vi "Actor Core.vi"(8 "error in":errorcluster, 11 "Counter in":refnum<class "Counter.lvclass">) -> (0 "error out":errorcluster, 3 "Actor out":refnum<class "Actor.lvclass">)   [LabVIEW 2013, in "Counter.lvclass"]
doc: "(<B>Filename</B>: Actor Framework.lvlib:Actor.lvclass:Actor Core.vi)\n\nReceives messages to the actor, reacts to them, and initiates any error handling that may shut the actor down.\n\nDescendant classes may override this VI to append parallel tasks for the actor to complete while it handles messages. Overrides use the Call Parent Method node."
uses:
  Counter.lvclass
  <vilib>/ActorFramework/Actor/Actor.lvclass
  Display.lvclass/DisplayUI.lvclass
  <vilib>/ActorFramework/Actor/Actor.lvclass/Actor.ctl
  <vilib>/ActorFramework/Message Enqueuer/Message Enqueuer.lvclass/Message Enqueuer.ctl
  Counter.lvclass/Counter.ctl
  <vilib>/ActorFramework/Message Enqueuer/Init from Existing Queue.vi
  <vilib>/ActorFramework/Message Enqueuer/Enqueue.vi
  <vilib>/ActorFramework/Message Priority Queue/Priority Enqueue.vi
  <vilib>/ActorFramework/Message Enqueuer/Message Enqueuer.lvclass
  <vilib>/ActorFramework/Stop Msg/Stop Msg.lvclass
  Counter Messages/CountZero Msg/CountZero Msg.lvclass
  Counter Messages/DataToDisplay Msg/DataToDisplay Msg.lvclass
panel:
  in  "ToZero":bool
  in  "Exit":bool
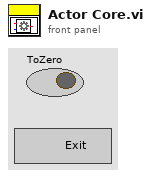
[diagram p1: front panel]
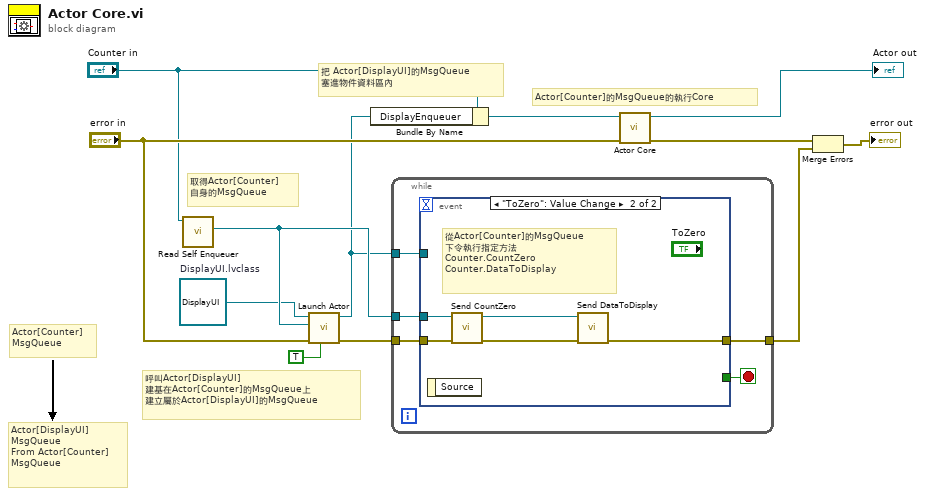
[diagram p0: block diagram]
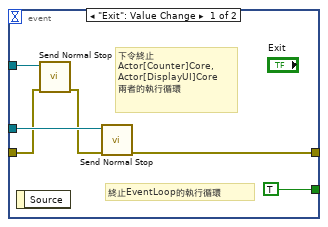
[diagram p2: hidden frame]
diagram:
  w1 = refnum<class "DisplayUI.lvclass"> refnum  # DisplayUI.lvclass
  # "Actor[DisplayUI]\nMsgQueue\nFrom Actor[Counter]\nMsgQueue"
  # "Actor[Counter]\nMsgQueue"
  # "Actor[Counter]的MsgQueue的執行Core"
  # "把 Actor[DisplayUI]的MsgQueue\n塞進物件資料區內"
  # "呼叫Actor[DisplayUI]\n建基在Actor[Counter]的MsgQueue上\n建立屬於Actor[DisplayUI]的MsgQueue"
  # "取得Actor[Counter]\n自身的MsgQueue"
  n1 = call <vilib>:"Read Self Enqueuer.vi"("Actor"="Counter in") -> ("Self Enqueuer"=w7:refnum<class "Message Enqueuer.lvclass">)  [unwired: 10 in]
  n2 = call <vilib>:"Launch Actor.vi"("Open Actor Core front panel? (F)"=TRUE, "error in (no error)"="error in", "Actor-to-Caller Enqueuer"=w7, "Actor"=w1) -> ("error out"=w6:errorcluster, "Caller-To-Actor Enqueuer"=w2:refnum<class "Message Enqueuer.lvclass">)  [unwired: 6 in]
  n3 = Bundle By Name(cluster="Counter in", "DisplayEnqueuer"=w2) -> (w3:refnum<class "Counter.lvclass">)
  n4 = while {
    tunnel: w7 -> [w16]
    tunnel: w6 -> [w15]
    tunnel: [w14] -> w8
    tunnel: w2 -> [w13]
    stop <- w17 stop-if-true
    n5 = event shown="[1] \"ToZero\": Value Change" {
      selector: _ -> [_ _]
      dyn-events: _ -> [_ _]
      timeout: _ -> [_ _]
      tunnel: [TRUE _] -> w17
      tunnel: w16 -> [w22 w28]
      tunnel: w15 -> [w19 w25]
      tunnel: [w21 w24] -> w14
      tunnel: w13 -> [w20 _]
      event "Exit": Value Change {
        # "終止EventLoop的執行循環"
        # "下令終止\nActor[Counter]Core,\nActor[DisplayUI]Core\n兩者的執行循環"
        n6 = event-data() -> ()  [unwired: 1 in, 1 out]
        n7 = call <vilib>:"Send Normal Stop.vi"("error in (no error)"=w19, "Message Enqueuer"=w20) -> ("error out"=w18:errorcluster)  [unwired: 9 in]
        n8 = call <vilib>:"Send Normal Stop.vi"("error in (no error)"=w18, "Message Enqueuer"=w22) -> ("error out"=w21:errorcluster)  [unwired: 9 in]
      }
      event "ToZero": Value Change {
        # "從Actor[Counter]的MsgQueue\n下令執行指定方法\nCounter.CountZero\nCounter.DataToDisplay"
        n9 = event-data() -> ()  [unwired: 1 in, 1 out]
        n10 = call "Send CountZero.vi"("error in (no error)"=w25, "Message Enqueuer"=w28) -> ("error out"=w26:errorcluster, "Message Enqueuer out"=w27:refnum<class "Message Enqueuer.lvclass">)  [unwired: 8 in]
        n11 = call "Send DataToDisplay.vi"("error in (no error)"=w26, "Message Enqueuer"=w27) -> ("error out"=w24:errorcluster)  [unwired: 8 in, 1 out]
      }
    }
  }
  n12 = call-parent "Actor Core.vi"("error in"="error in", "Actor in"=w3) -> ("error out"=w12:errorcluster, "Actor out"=→"Actor out":refnum<class "Actor.lvclass">)  [unwired: 8 in]
  n13 = Merge Errors(w12, w8) -> (→"error out":errorcluster)
